vi "Scripting.vi"() -> ()   [LabVIEW 2019]
doc: "This example demonstrates how to make an existing VI into a type defition. It is important to understand that a type definition is a special type of VI. Therefore, you need to create a VI of type, \"Control VI\" first. By default, a control VI is template for a custom control, not a type definition. You must change the control VI type to typedef using a VI Property node.\n\nIn this example, a control is copied from a standard VI, called \"VIToModify\" using the StyleID property node. This is the control that will be made into a type definition. Then a type definition VI is created, and the control is added using the styleID. Then, the control on VIToModify is replaced with the type definition that was just created. \n\nNote: Scripting is included with LabVIEW 2012. No extra download or activation is needed. Simply enable in your Tools>>Options Dialog."
uses:
  <vilib>/Utility/miscctls.llb/LVPointTypeDef.ctl
panel:
  out "Error Out":errorcluster
  in  "VI name":string="VIToModify.vi"
  in  "Control name":string="awesome.ctl"
  # "Notes: the file directory is set to the\nlocation of the Scripting.vi directory.\nThe control name must have a .ctl\nextension and the VI name must have\na .vi extension."
  # "The Control name is the type definition control that is created. \nThe VI name is the the VI that already exists, where the existing\ncontrol properties are taken from."
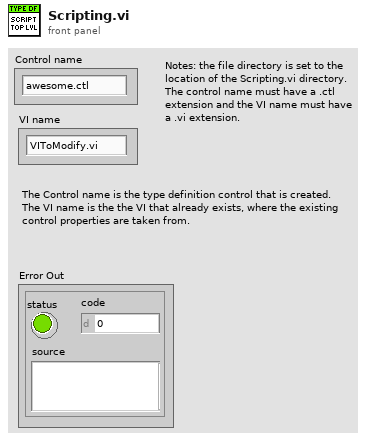
[diagram p1: front panel]
types:
  T1 = enum32{"not a control VI", "control", "typedef", "strict typedef"}
  T2 = typedef "LVPointTypeDef.ctl" = cluster{"Horizontal":i16, "Vertical":i16}
  T3 = enum32{"invalid VI type", "Standard VI", "Control VI", "Global VI", "Polymorphic VI", "Configuration VI", "SubSystem", "Facade VI", "Method VI", "Statechart Diagram VI"}
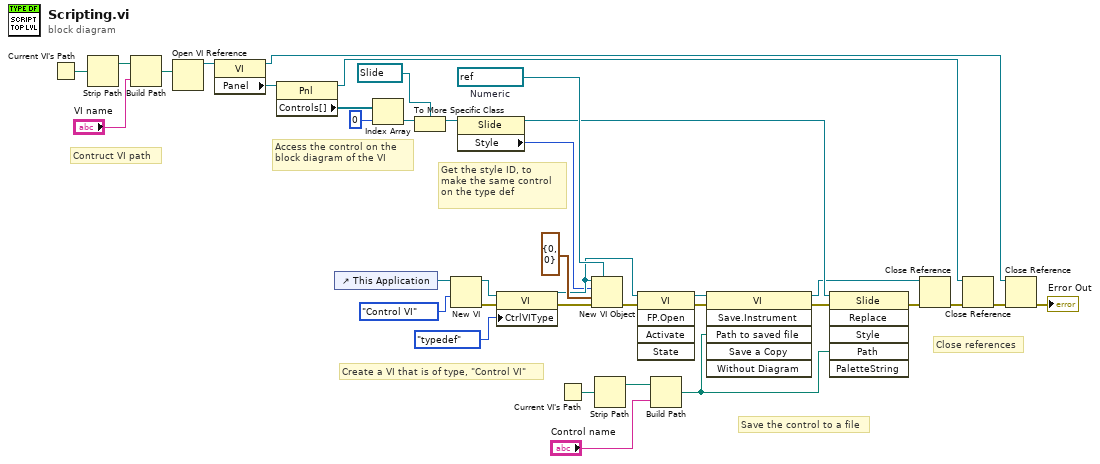
[diagram p0: block diagram]
diagram:
  w32 = refnum<vi> refnum  # Numeric
  # "Close references"
  # "Save the control to a file"
  # "Create a VI that is of type, \"Control VI\""
  # "Get the style ID, to\nmake the same control \non the type def"
  # "Access the control on the \nblock diagram of the VI"
  # "Contruct VI path"
  n1 = Current VI's Path() -> (path=w11:path)
  n2 = Strip Path(path=w11) -> (stripped path=w10:path)  [unwired: 1 out]
  n3 = Build Path(base path=w10, name or relative path="VI name") -> (appended path=w8:path)
  n4 = Open VI Reference(vi path=w8) -> (vi reference=w18:refnum<vi>)  [unwired: 5 in, 1 out]
  n5 = property class="VI"(reference=w18) -> (reference out=w4:refnum<vi>, "Panel"=w35:refnum<vi>)  [unwired: 1 in, 1 out]
  n6 = property class="Pnl"(reference=w35) -> (reference out=w6:refnum<vi>, "Controls[]"=w37:refnum<vi>[])  [unwired: 1 in, 1 out]
  n7 = control-ref of="This Application"() -> (w33:refnum<vi>)
  n8 = Index Array(array=w37, index=0) -> (element=w20:refnum<vi>)
  n9 = To More Specific Class(target class=refnum<vi> refnum ("reference"), reference=w20) -> (specific class reference=w19:refnum<vi>)  [unwired: 1 in, 1 out]
  n10 = New VI(9:T3."Control VI" ("vi type (standard vi)"), 11:w33) -> (0:w27:errorcluster, 3:w24:refnum<vi>)  [unwired: 5 in]
  n11 = property on="Property Node" class="Slide"(reference=w19) -> (reference out=w17:refnum<vi>, "Style"=w25:u32)  [unwired: 1 in, 1 out]
  n12 = property class="VI"(reference=w24, error in=w27, "CtrlVIType"=T1."typedef" ("Control VI Type")) -> (reference out=w28:refnum<vi>, error out=w26:errorcluster)
  n13 = Current VI's Path() -> (path=w15:path)
  n14 = New VI Object(vi object class=w32, owner refnum=w28, style=w25, position/next to=T2 {"Horizontal"=0, "Vertical"=0} ("location"), 8:w26) -> (0:w30:errorcluster)  [unwired: 3 in, 1 out]
  n15 = Strip Path(path=w15) -> (stripped path=w14:path)  [unwired: 1 out]
  n16 = invoke class="VI" method="FP.Open"(reference=w28, error in=w30) -> (reference out=w21:refnum<vi>, error out=w23:errorcluster)  [unwired: 3 in, 3 out]
  n17 = Build Path(base path=w14, name or relative path="Control name") -> (appended path=w13:path)
  n18 = invoke class="VI" method="Save.Instrument"(reference=w21, error in=w23, "Path to saved file"=w13) -> (reference out=w2:refnum<vi>, error out=w16:errorcluster)  [unwired: 3 in, 4 out]
  n19 = invoke on="Invoke Node" class="Slide" method="Replace"(reference=w17, error in=w16, "Path"=w13) -> (error out=w1:errorcluster)  [unwired: 3 in, 5 out]
  n20 = Close Reference(reference=w2, error in (no error)=w1) -> (error out=w7:errorcluster)
  n21 = Close Reference(reference=w6, error in (no error)=w7) -> (error out=w5:errorcluster)
  n22 = Close Reference(reference=w4, error in (no error)=w5) -> (error out=→"Error Out":errorcluster)
